vi "Version 1_Legacy Detector.vi"(7 "Address (A)":string="A", 8 "error in":errorcluster, 11 "VISA Session In":refnum<visa-resource-name>="Alicat") -> (0 "error out":errorcluster, 1 "Legacy Unit?":enum32{"32-Bit Unit", "16-bit Unit"}(radio), 3 "VISA Session Out":refnum<visa-resource-name>)   [LabVIEW 2016]
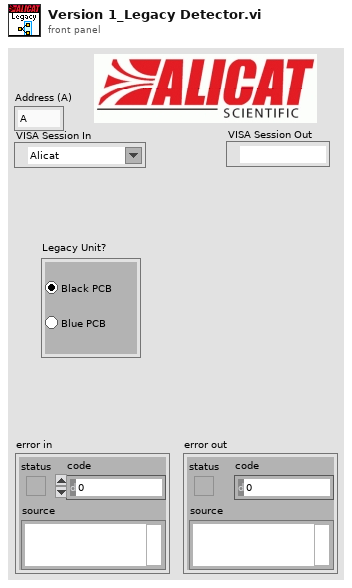
[diagram p1: front panel]
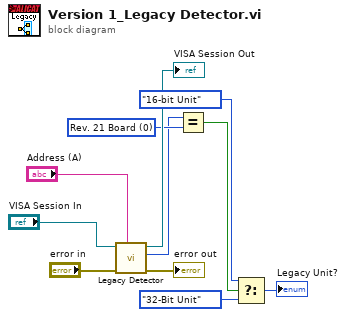
[diagram p0: block diagram]
diagram:
  w6 = u8 0 items=["Rev. 21 Board", "Rev. 22 Board", "Rev. 23 Board"] ("Legacy Status")
  n1 = call "Legacy Detector.vi"("Unit ID (A)"="Address (A)", "error in"="error in", "VISA Session In"="VISA Session In") -> ("error out"=→"error out":errorcluster, "Legacy Status"=w5:u8, "VISA Session Out"=→"VISA Session Out":refnum<visa-resource-name>)  [unwired: 6 in]
  n2 = Equal?(x=w5, y=w6) -> (x = y?=w4:bool)
  n3 = Select(t=enum32{"32-Bit Unit", "16-bit Unit"}."16-bit Unit" ("Legacy Unit?"), s=w4, f=enum32{"32-Bit Unit", "16-bit Unit"}."32-Bit Unit" ("Legacy Unit?")) -> (s? t:f=→"Legacy Unit?":enum32{"32-Bit Unit", "16-bit Unit"})
